vi "시분초파일 하다맘.vi"() -> ()   [LabVIEW 2014]
panel:
  out "날짜/시간 문자열":string
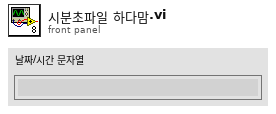
[diagram p1: front panel]
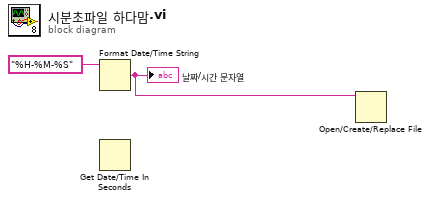
[diagram p0: block diagram]
diagram:
  n1 = Format Date/Time String(time format string (%c)="%H-%M-%S" ("시간 포맷 문자열 (%c)")) -> (date/time string=w1:string)  [unwired: 2 in]
  "날짜/시간 문자열" <- w1
  n2 = Get Date/Time In Seconds() -> ()  [unwired: 1 out]
  n3 = Open/Create/Replace File(file path (use dialog)=w1) -> ()  [unwired: 5 in, 3 out]
